vi "DB_EscribeTablaAlarmas.vi"(8 "error in (no error)":errorcluster, 10 "MOTIVO":string, 11 "ID_EQUIPO":i32) -> (0 "error out":errorcluster)   [LabVIEW 2018]
uses:
  <vilib>/addons/database/Connection.llb/DB Tools Open Connec (Path).vi
  <vilib>/addons/database/Connection.llb/Conn Execute.vi
  <vilib>/addons/database/Recordset.llb/Rec Destroy - Connection.vi
  <vilib>/addons/database/NI_Database_API.lvlib
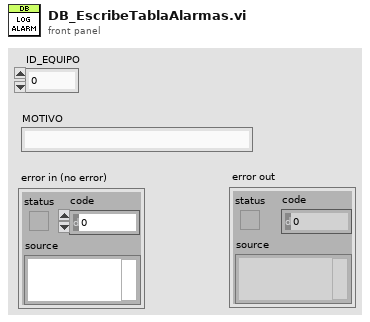
[diagram p1: front panel]
types:
  T1 = typedef "NI_Database_API.lvlib/Conn ObjectReference.ctl" = refnum<k1>
  T2 = typedef "NI_Database_API.lvlib/Rec ObjectReference.ctl" = refnum<k1>
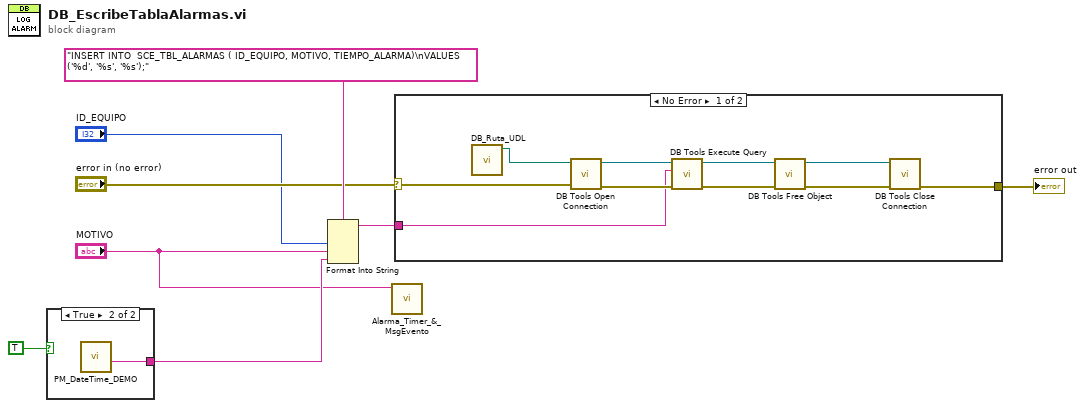
[diagram p0: block diagram]
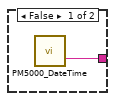
[diagram p2: hidden frame]
diagram:
  n1 = case shown="True" TRUE {
    tunnel: [w9 w10] -> w3
    frame False {
      n2 = call "PM5000_DateTime.vi"() -> ("TIEMPO_MEDICION"=w9:string)  [unwired: 8 in, 3 out]
    }
    frame True {
      n3 = call "PM_DateTime_DEMO.vi"() -> ("TIEMPO_MEDICION"=w10:string)  [unwired: 10 in, 1 out]
    }
  }
  n4 = Format Into String(format string="INSERT INTO  SCE_TBL_ALARMAS ( ID_EQUIPO, MOTIVO, TIEMPO_ALARMA)\nVALUES ('%d', '%s', '%s');" ("SQL"), "ID_EQUIPO", "MOTIVO", w3) -> (resulting string=w8:string)  [unwired: 2 in, 1 out]
  n5 = call "Alarma_Timer_&_MsgEvento.vi"("MOTIVO"="MOTIVO") -> ()  [unwired: 11 in]
  n6 = case shown="No Error" "error in (no error)" {
    selector: "error in (no error)" -> [w13 w21]
    tunnel: w8 -> [w17 _]
    tunnel: [w14 w21] -> w6
    frame No Error {
      n7 = call "DB_Ruta_UDL.vi"() -> ("UDL ruta"=w12:path)  [unwired: 11 in]
      n8 = call-poly <vilib>:"DB Tools Open Connection.vi"("error in (no error)"=w13, "connection information"=w12) -> ("error out"=w20:errorcluster, "connection reference"=w18:T1)  [unwired: 6 in]
      n9 = call-poly <vilib>:"DB Tools Execute Query.vi"("error in (no error)"=w20, "SQL query"=w17, "connection reference"=w18) -> ("error out"=w19:errorcluster, "recordset reference"=w15:T2)  [unwired: 5 in]
      n10 = call-poly <vilib>:"DB Tools Free Object.vi"("error in (no error)"=w19, "recordset reference"=w15) -> ("error out"=w16:errorcluster, "connection reference"=w11:T1)  [unwired: 8 in]
      n11 = call <vilib>:"DB Tools Close Connection.vi"("error in (no error)"=w16, "connection reference"=w11) -> ("error out"=w14:errorcluster)  [unwired: 5 in]
    }
    frame Error {
    }
  }
  "error out" <- w6
